vi "_Read (No Objects).vi"(8 "error in (no error)":errorcluster, 11 "Cluster In":T3={"helium"={"fastHe?"=FALSE, "slowHe?"=FALSE, "fillHe?"=FALSE, "lowHe?"=FALSE}, "nitrogen"={"fillN?"=FALSE, "lowN?"=FALSE}, "Shutdown"=FALSE, "Cryogen Levels"=[], "IO Info"={"Address"={"Com Port"=1, "ISOBUS Address"=5, "GPIB Address"=24, "Communication"=enum."ISOBUS"}, "ILM Name"="", "Display Channel"=[]}} {"Cryogen Levels" min=-1.0 max=100.0 scale=0.0..100.0}) -> (0 "error out":errorcluster, 2 "X array":T4, 3 "Cluster Out":T3={"helium"={"fastHe?"=FALSE, "slowHe?"=FALSE, "fillHe?"=FALSE, "lowHe?"=FALSE}, "nitrogen"={"fillN?"=FALSE, "lowN?"=FALSE}, "Shutdown"=FALSE, "Cryogen Levels"=[], "IO Info"={"Address"={"Com Port"=1, "ISOBUS Address"=5, "GPIB Address"=24, "Communication"=enum."ISOBUS"}, "ILM Name"="", "Display Channel"=[]}} {"Cryogen Levels" min=-1.0 max=100.0 scale=0.0..100.0})   [LabVIEW 2009]
doc: "(Protected, Dynamic, Pure Virtual/Abstract) Perform a measurement and return one or more channels of data. Outsiders should not call this method, but instead the public \"Read Data.vi\"."
uses:
  Utility Classes/Readable/X array.ctl
  Utility Classes/Readable/X.ctl
  Cryogen Levels.ctl
  Oxford/BUSGEN.LLB/OxfordAddress.ctl
  Utility Classes/Readable/Readable.lvclass
  Level Meter.lvclass
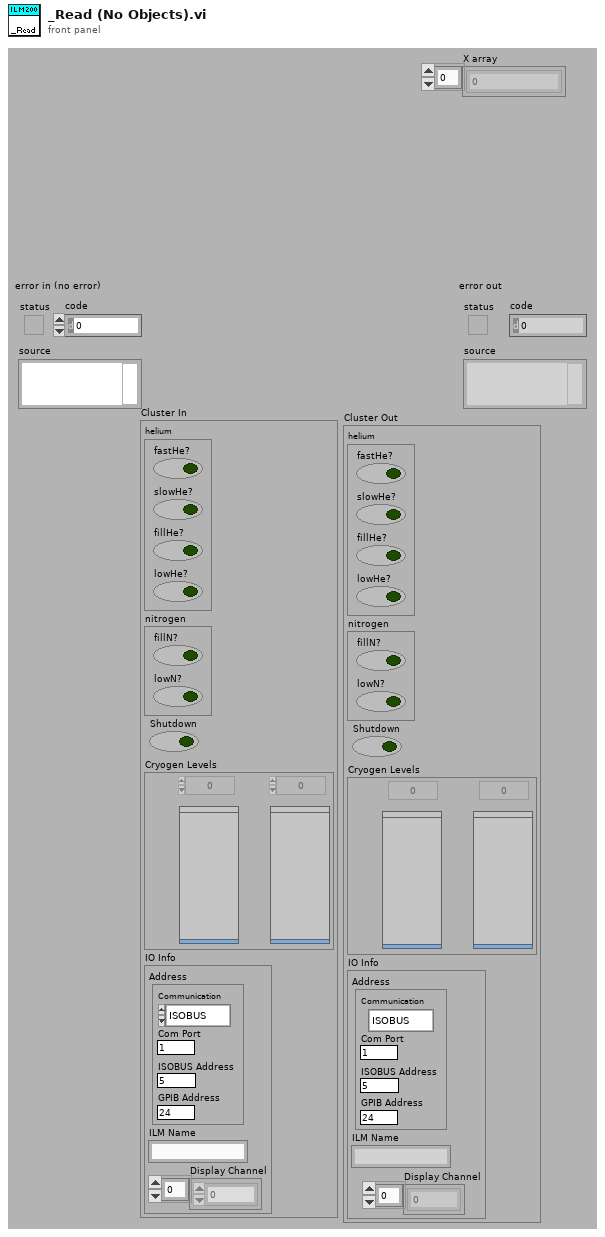
[diagram p1: front panel]
types:
  T1 = typedef "Level Meter.lvclass/Cryogen Levels.ctl" = dbl[]
  T2 = typedef "OxfordAddress.ctl" = cluster{"Com Port":i32, "ISOBUS Address":i32, "GPIB Address":i16, "Communication":enum16{"RS232", "ISOBUS", "GPIB", "Gateway"}}
  T3 = cluster{"helium":cluster{"fastHe?":bool, "slowHe?":bool, "fillHe?":bool, "lowHe?":bool}, "nitrogen":cluster{"fillN?":bool, "lowN?":bool}, "Shutdown":bool, "Cryogen Levels":T1, "IO Info":cluster{"Address":T2, "ILM Name":string, "Display Channel":i32[]}}
  T4 = typedef "Readable.lvclass/X array.ctl" = T5[]
  T5 = typedef "Readable.lvclass/X.ctl" = dbl
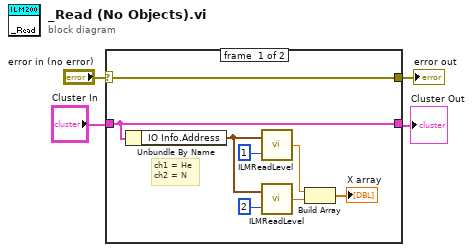
[diagram p0: block diagram]
diagram:
  n1 = case shown="No Error" "error in (no error)" {
    selector: "error in (no error)" -> [w5 w14]
    tunnel: "Cluster In" -> [w6 w13]
    tunnel: [w6 w13] -> w1
    tunnel: [w5 w14] -> w3
    frame #0 {
      # "ch1 = He\nch2 = N"
      n2 = Unbundle By Name(w6) -> ("IO Info.Address"=w10:T2)
      n3 = call "ILMReadLevel.vi"("Address"=w10, "Channel number (1-3)"=1) -> ("Level"=w9:dbl)  [unwired: 2 out]
      n4 = call "ILMReadLevel.vi"("Address"=w10, "Channel number (1-3)"=2) -> ("Level"=w7:dbl)  [unwired: 2 out]
      n5 = Build Array(w9, w7) -> (→"X array":dbl[])
    }
    frame #1 {
    }
  }
  "error out" <- w3
  "Cluster Out" <- w1
